vi "Discover Signal Generator Model.vi"(10 "Model In":string) -> (2 "selection":bool)   [LabVIEW 2018]
panel:
  out "size(s)":i32
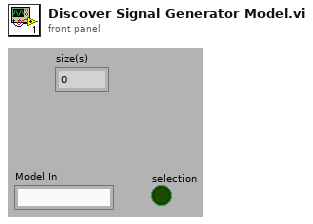
[diagram p1: front panel]
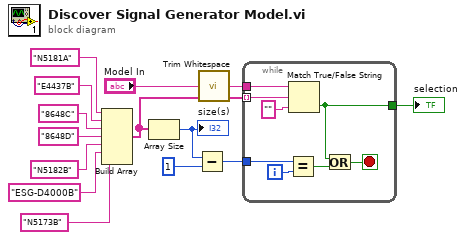
[diagram p0: block diagram]
diagram:
  n1 = Build Array("N5181A" ("element"), "E4437B" ("true string"), "8648C" ("true string"), "8648D" ("true string"), "N5182B" ("true string"), "ESG-D4000B" ("true string"), "N5173B" ("element")) -> (w12:string[])
  n2 = Array Size(array=w12) -> (size(s)=w11:i32)
  "size(s)" <- w11
  n3 = Subtract(x=w11, y=1) -> (x-y=w9:i32)
  n4 = call <vilib>:"Trim Whitespace.vi"("string"="Model In") -> ("trimmed string"=w7:string)  [unwired: 1 in]
  n5 = while {
    tunnel: w12 -> [w21] mode=indexing
    tunnel: w7 -> [w20]
    tunnel: [w19] -> w13
    tunnel: w9 -> [w15]
    i -> [w16]
    stop <- w18 stop-if-true
    n6 = Equal?(x=w15, y=w16) -> (x = y?=w17:bool)
    n7 = Match True/False String(2:"" ("false string"), 3:w21, 4:w20) -> (0:w19:bool)  [unwired: 1 out]
    n8 = Or(x=w19, y=w17) -> (x .or. y?=w18:bool)
  }
  "selection" <- w13
